vi "whilefor2.vi"() -> ()   [LabVIEW 2022 SP3]
panel:
  in  "Limit":i32 format="%#.0g"
  in  "stop":bool
  out "end of loop":bool
  out "current value of iterator":dbl
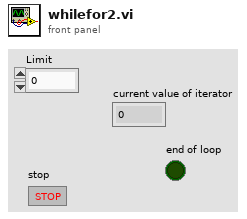
[diagram p1: front panel]
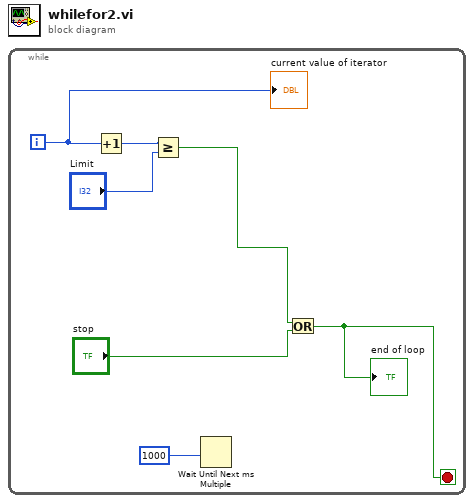
[diagram p0: block diagram]
diagram:
  n1 = while {
    i -> [w3]
    stop <- w6 stop-if-true
    n2 = Increment(x=w3) -> (x+1=w2:i32)
    n3 = Greater Or Equal?(x=w2, y="Limit") -> (x >= y?=w4:bool)
    n4 = Wait Until Next ms Multiple(millisecond multiple=1000) -> ()  [unwired: 1 out]
    n5 = Or(x=w4, y="stop") -> (x .or. y?=w6:bool)
    "end of loop" <- w6
    "current value of iterator" <- w3
  }
